vi "demo.vi"(0 "reference (in)":i32, 1 "position ref":refnum<vi>, 2 "position (large) ref":refnum<vi>, 5 "positions":i32[](array[numeric]), 11 "error in (no error)":errorcluster, 12 "Current State (display)":refnum<vi>, 13 "status":refnum<vi>) -> (4 "reference (out)":i32, 15 "error out":errorcluster)   [LabVIEW 2012]
doc: "Cycles the motor to each position in the input array of positions.\n\nProduced by:\n\nChristopher Lemieux\nTest and Automation Engineer\ntestengnr@yahoo.com"
uses:
  main_functions/commands.ctl
  utilities/getters/controls/status_states.ctl
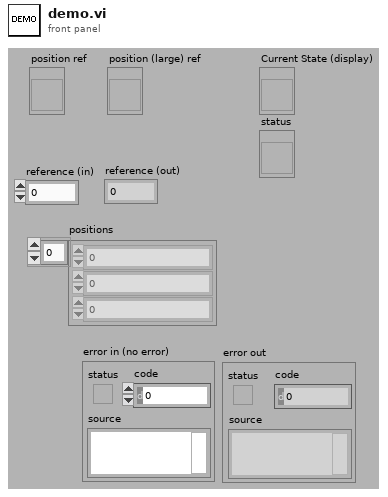
[diagram p1: front panel]
types:
  T1 = typedef "commands.ctl" = enum16{"clear error", "constant jog(-)", "constant jog(+)", "get acceleration", "get actual current", "get device id", "get digital input status", "get digial inputs status", "get dig output status", "get digital outputs status", "get firmware ver", "get high speed", "get idle current", "get low speed", "get micro step", "get motor status", "get move mode", "get polarity", "get position", "get product id", "get power status", "get run current", "get status", "home(-)", "home(+)", "move to position", "power down", "power up", "set acceleration", "set device id", "set digital output", "set digital outputs", "set high speed", "set idle current", "set low speed", "set move mode absolute", "set move mode increment", "set polarity", "set position", "set run current", "stop immediate", "stop slow", "store to memory"}
  T2 = typedef "status_states.ctl" = enum16{"IDLE", "CONST", "ACCEL", "DECEL", "HOME_SWITCH", "-LIMIT_SWITCH", "+LIMIT_SWITCH", "-LIMIT_ERR", "+LIMIT_ERR", "COMM_ERR"}
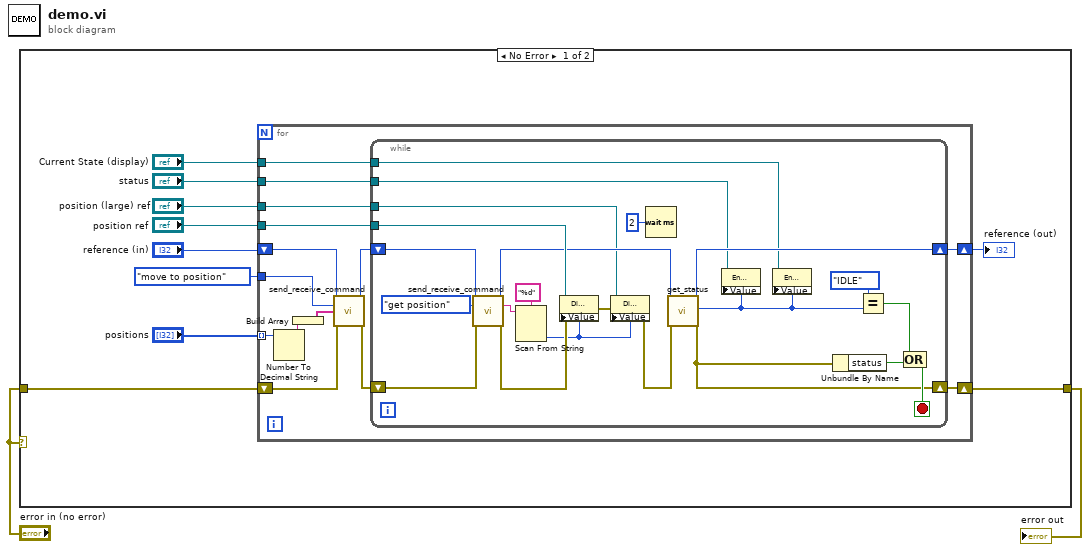
[diagram p0: block diagram]
diagram:
  n1 = case shown="No Error" "error in (no error)" {
    tunnel: "error in (no error)" -> [w8 w49]
    tunnel: [w7 w49] -> w1
    frame No Error {
      n2 = for {
        shift-right: [w20] -> w7
        shift-left: w8 -> [w21]
        tunnel: "positions" -> [w18] mode=indexing
        shift-right: [w24] -> w9
        shift-left: "reference (in)" -> [w26]
        tunnel: "position ref" -> [w23]
        tunnel: commands."move to position" ("commands") -> [w19]
        tunnel: "position (large) ref" -> [w15]
        tunnel: "Current State (display)" -> [w14]
        tunnel: "status" -> [w13]
        n3 = Number To Decimal String(number=w18) -> (decimal integer string=w17:string)  [unwired: 1 in]
        n4 = Build Array(w17) -> (w16:string[])
        n5 = call "send_receive_command.vi"("reference (in)"=w26, "command"=w19, "params (opt)"=w16, "error in (no error)"=w21) -> ("reference (dup)"=w25:i32, "error out"=w22:errorcluster)  [unwired: 7 in, 3 out]
        n6 = while {
          shift-right: [w47] -> w24
          shift-left: w25 -> [w39]
          tunnel: w23 -> [w42]
          shift-right: [w37] -> w20
          shift-left: w22 -> [w41]
          tunnel: w15 -> [w33]
          tunnel: w14 -> [w29]
          tunnel: w13 -> [w28]
          stop <- w45 stop-if-true
          n7 = call "send_receive_command.vi"("reference (in)"=w39, "command"=commands."get position" ("commands"), "error in (no error)"=w41) -> ("reference (dup)"=w38:i32, "read_string"=w43:string, "error out"=w40:errorcluster)  [unwired: 8 in, 2 out]
          n8 = Scan From String(format string="%d", input string=w43) -> (output 1=w30:i32)  [unwired: 3 in, 3 out]
          n9 = property class="DigNum (strict)"(reference=w42, error in=w40, "Value"=w30) -> (error out=w32:errorcluster)  [unwired: 1 out]
          n10 = property class="DigNum (strict)"(reference=w33, error in=w32, "Value"=w30) -> (error out=w31:errorcluster)  [unwired: 1 out]
          n11 = Wait (ms)(milliseconds to wait=u32 2) -> ()  [unwired: 1 out]
          n12 = call "get_status.vi"("reference (in)"=w38, "error in (no error)"=w31) -> ("reference (dup)"=w47:i32, "motion_state"=w27:T2, "error out"=w37:errorcluster)  [unwired: 13 in, 2 out]
          n13 = property class="Enum (strict)"(reference=w28, "Value"=w27) -> ()  [unwired: 1 in, 2 out]
          n14 = property class="Enum (strict)"(reference=w29, "Value"=w27) -> ()  [unwired: 1 in, 2 out]
          n15 = Unbundle By Name(w37) -> ("status"=w46:bool)
          n16 = Equal?(x=status_states."IDLE", y=w27) -> (x = y?=w34:bool)
          n17 = Compound Arithmetic op=OR(w34, w46) -> (w45:bool)
        }
      }
      "reference (out)" <- w9
    }
    frame Error {
    }
  }
  "error out" <- w1
